vi "Write Enums As String.vi"(8 "error in (no error)":errorcluster, 10 "Enums As String (F)":bool, 11 "Serializer.JSON in":refnum<class "Serializer.JSON.lvclass">) -> (0 "error out":errorcluster, 3 "Serializer.JSON out":refnum<class "Serializer.JSON.lvclass">)   [LabVIEW 2019, in "OpenSerializer.JKI-JSON.lvlib" / "Serializer.JSON.lvclass"]
uses:
  Serializer.JSON.lvclass
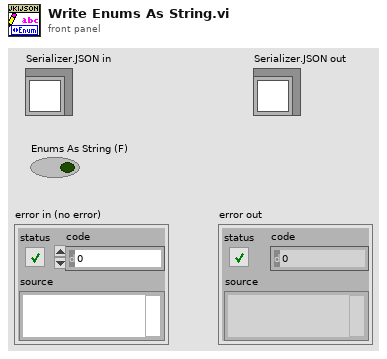
[diagram p1: front panel]
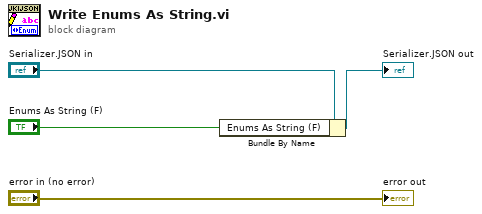
[diagram p0: block diagram]
diagram:
  n1 = Bundle By Name(cluster="Serializer.JSON in", "Enums As String (F)"="Enums As String (F)") -> (→"Serializer.JSON out":refnum<class "Serializer.JSON.lvclass">)
  "error out" <- "error in (no error)"
